vi "Generate_PRBS_Signal.vi"(9 "Min.Value":dbl, 10 "Max. Value":dbl, 11 "PRBS Order":i32) -> (2 "PRBS Signal Length":dbl, 3 "PRBS Signal":dbl[](array[numeric]))   [LabVIEW 2016]
uses:
  <vilib>/Analysis/NI_AALBase.lvlib
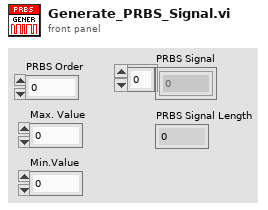
[diagram p1: front panel]
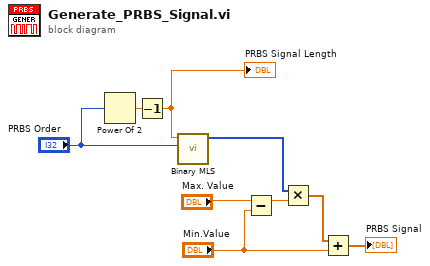
[diagram p0: block diagram]
diagram:
  n1 = Power Of 2(x="PRBS Order") -> (2^x=w8:dbl)
  n2 = Decrement(x=w8) -> (x-1=w9:dbl)
  "PRBS Signal Length" <- w9
  n3 = call <vilib>:"Binary MLS.vi"("polynomial order"="PRBS Order", "samples"=w9) -> ("mls sequence"=w5:u8[])  [unwired: 8 in, 1 out]
  n4 = Subtract(x="Max. Value", y="Min.Value") -> (x-y=w4:dbl)
  n5 = Multiply(x=w5, y=w4) -> (x*y=w2:dbl[])
  n6 = Add(x=w2, y="Min.Value") -> (x+y=→"PRBS Signal":dbl[])
